vi "windows_file.vi"(7 "operation":enum16{"open", "close", "read", "write"}(ring), 9 "string_in":string, 10 "FileName":string="\\\\.\\pipe\\cpc_out", 11 "handle_in":u32) -> (1 "string_out":string, 3 "handle_out":i32)   [LabVIEW 2018]
doc: "MeasGUI - Measurement Graphics User Interface\nCopyright (c) 2018 Frans Korhonen\n\nMeasGUI was originally developed at Institute for Atmospheric \nand Earth System Research / Physics, Faculty of Science, \nUniversity of Helsinki, Finland\n\nAssistance, experience and feedback from following persons have been \ncritical in development of MeasGUI: Michel Attoui, Juha Kangasluoma, \nLauri Ahonen, Ella Häkkinen, Markku Kulmala and Tuukka Petäjä.\n\nThis file is part of MeasGUI.\n\nThis Source Code Form is subject to the terms of the Mozilla Public\nLicense, v. 2.0. If a copy of the MPL was not distributed with this\nfile, You can obtain one at http://mozilla.org/MPL/2.0/."
uses:
  kernel32.dll
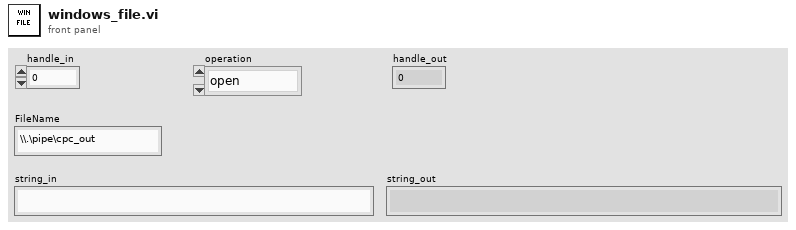
[diagram p1: front panel]
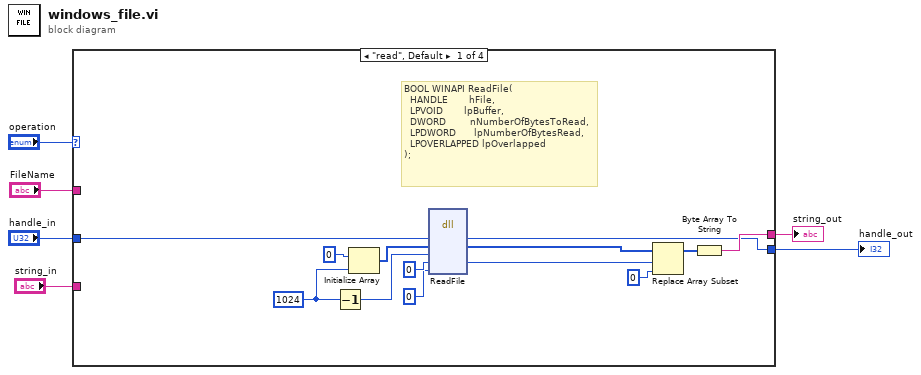
[diagram p0: block diagram]
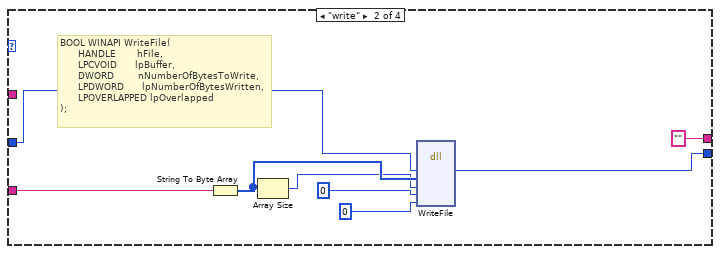
[diagram p2: hidden frame]
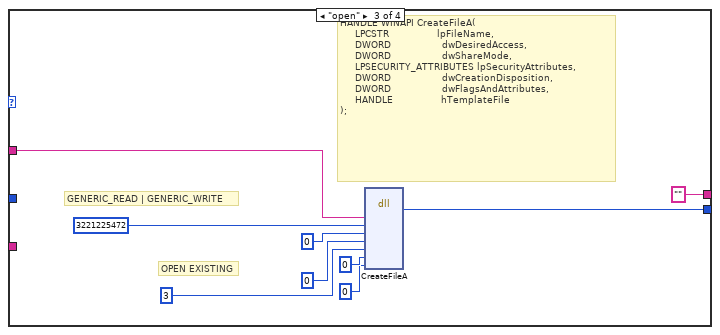
[diagram p3: hidden frame]
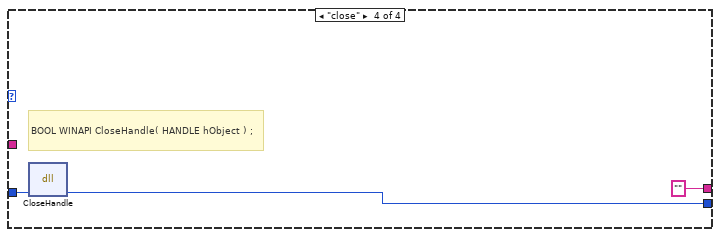
[diagram p4: hidden frame]
diagram:
  n1 = case shown="\"read\", Default" "operation" {
    tunnel: "FileName" -> [_ _ w31 _]
    tunnel: [w7 w22 w29 w38] -> w5
    tunnel: "handle_in" -> [w17 w23 _ w39]
    tunnel: [w10 "" ("string") "" ("string") "" ("string")] -> w2
    tunnel: "string_in" -> [_ w26 _ _]
    frame "read", Default {
      w15 = 1024 ("dimension size")
      # "BOOL WINAPI ReadFile(\n  HANDLE       hFile,\n  LPVOID       lpBuffer,\n  DWORD        nNumberOfBytesToRead,\n  LPDWORD      lpNumberOfBytesRead,\n  LPOVERLAPPED lpOverlapped\n);"
      n2 = Decrement(x=w15) -> (x-1=w13:i32)
      n3 = Initialize Array(u8 0, w15) -> (w14:u8[])
      n4 = dll-call lib="kernel32.*" fn="ReadFile"("hFile"=w17, "lpBuffer"=w14, "nNumberOfBytesToRead"=w13, "lpNumberOfBytesRead"=u32 0, "lpOverlapped"=u32 0) -> ("hFile"=w7:u32, "lpBuffer"=w9:u8[], "lpNumberOfBytesRead"=w8:u32)  [unwired: 6 in, 2 out]
      n5 = Replace Array Subset(array=w9, new element=u8 0 ("new element/subarray"), index=w8) -> (w11:u8[])
      n6 = Byte Array To String(unsigned byte array=w11) -> (string=w10:string)
    }
    frame "write" {
      # "BOOL WINAPI WriteFile(\n      HANDLE       hFile,\n      LPCVOID      lpBuffer,\n      DWORD        nNumberOfBytesToWrite,\n      LPDWORD      lpNumberOfBytesWritten,\n      LPOVERLAPPED lpOverlapped\n);"
      n7 = String To Byte Array(string=w26) -> (unsigned byte array=w21:u8[])
      n8 = Array Size(array=w21) -> (size(s)=w20:i32)
      n9 = dll-call lib="kernel32.*" fn="WriteFile"("hFile"=w23, "lpBuffer"=w21, "nNumberOfBytesToWrite"=w20, "lpNumberOfBytesWritten"=u32 0, "lpOverlapped"=u32 0) -> ("hFile"=w22:u32)  [unwired: 8 in, 2 out]
    }
    frame "open" {
      # "GENERIC_READ | GENERIC_WRITE"
      # "HANDLE WINAPI CreateFileA(\n     LPCSTR                lpFileName,\n     DWORD                 dwDesiredAccess,\n     DWORD                 dwShareMode,\n     LPSECURITY_ATTRIBUTES lpSecurityAttributes,\n     DWORD                 dwCreationDisposition,\n     DWORD                 dwFlagsAndAttributes,\n     HANDLE                hTemplateFile\n);"
      # "OPEN EXISTING"
      n10 = dll-call lib="kernel32.*" fn="CreateFileA"("lpFileName"=w31, "dwDesiredAccess"=u32 3221225472, "dwShareMode"=u32 0, "lpSecurityAttributes"=u32 0, "dwCreationDisposition"=u32 3 ("dwDesiredAccess"), "dwFlagsAndAttributes"=u32 0, "hTemplateFile"=u32 0) -> ("return type"=w29:u32)  [unwired: 10 in, 2 out]
    }
    frame "close" {
      # "BOOL WINAPI CloseHandle( HANDLE hObject ) ;"
      n11 = dll-call lib="kernel32.*" fn="CloseHandle"("hObject"=w39) -> ("hObject"=w38:u32)  [unwired: 4 in, 2 out]
    }
  }
  "handle_out" <- w5
  "string_out" <- w2
